vi "Get Events.vi"(11 "Duplicated Node Dialog View in":refnum<class "Duplicated Node Dialog View.lvclass">) -> (2 "Events":T1, 3 "Duplicated Node Dialog View out":refnum<class "Duplicated Node Dialog View.lvclass">)   [LabVIEW 2013, in "Duplicated Node Dialog View.lvlib" / "Duplicated Node Dialog View.lvclass"]
uses:
  Duplicated Node Dialog View.lvclass
  Typedef/Events.ctl
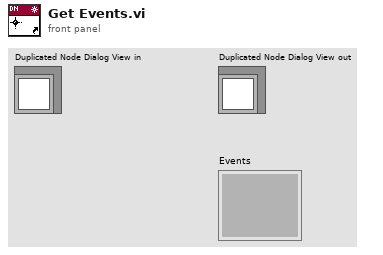
[diagram p1: front panel]
types:
  T1 = typedef "Duplicated Node Dialog View.lvlib/Duplicated Node Dialog View.lvclass/Events.ctl" = cluster{}
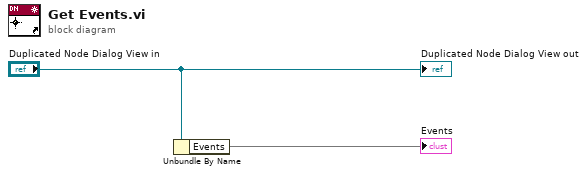
[diagram p0: block diagram]
diagram:
  n1 = Unbundle By Name("Duplicated Node Dialog View in") -> ("Events"=→"Events")
  "Duplicated Node Dialog View out" <- "Duplicated Node Dialog View in"
